vi "Pay.vi"(8 "error in (no error)":errorcluster, 10 "Amount":dbl, 11 "ACreditAccount in":refnum<class "ACreditAccount.lvclass">) -> (0 "error out":errorcluster, 2 "Balance":dbl, 3 "ACreditAccount out":refnum<class "ACreditAccount.lvclass">)   [LabVIEW 2020, in "ACreditAccount.lvclass"]
uses:
  ACreditAccount.lvclass
  ACreditAccount.lvclass/ACreditAccount.ctl
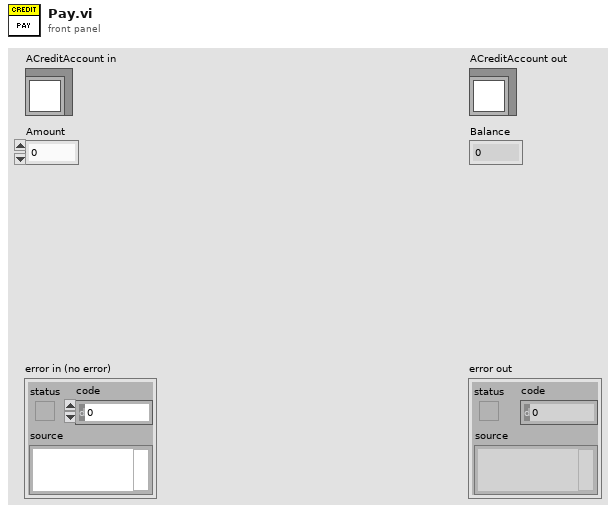
[diagram p1: front panel]
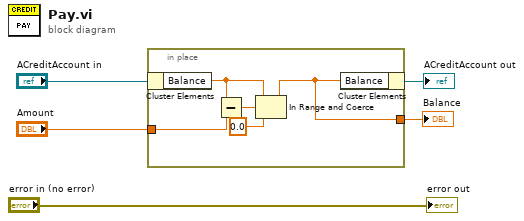
[diagram p0: block diagram]
diagram:
  n1 = in-place {
    in-place-border: "Amount" -> [w10]
    in-place-border: [w6] -> w2
    n2 = in-place-cluster #1("ACreditAccount in") -> ("Balance"=w8:dbl)
    n3 = Subtract(x=w8, y=w10) -> (x-y=w9:dbl)
    n4 = In Range and Coerce(upper limit=w8, x=w9, lower limit=0.0) -> (coerced(x)=w6:dbl)  [unwired: 1 out]
    n5 = in-place-cluster #1("Balance"=w6) -> (→"ACreditAccount out":refnum<class "ACreditAccount.lvclass">)
  }
  "Balance" <- w2
  "error out" <- "error in (no error)"
